vi "Write Notification Msg Return Info.vi"(8 "Return Priority (Normal)":T1=enum."Normal", 9 "Datum Name":string, 10 "Message Enqueuer in":refnum<class "Message Enqueuer.lvclass">, 11 "Notification Msg In":refnum<class "Notification Msg.lvclass">) -> (3 "Notification Msg Out":refnum<class "Notification Msg.lvclass">)   [LabVIEW 2017, in "Transport.lvlib" / "Notification Msg.lvclass"]
doc: "<License>\nCopyright © 2017 Composed Systems, LLC | All rights reserved\nwww.composed.io\n\nAuthor: Ethan Stern <ethan.stern@composed.io>\n\nThis software is provided \"AS IS\" WITHOUT WARRANTIES, either express or implied, AND IS FOR EDUCATIONAL PURPOSES ONLY.\n</License>"
uses:
  Notification Msg.lvclass
  <vilib>/ActorFramework/Message Enqueuer/Message Enqueuer.lvclass
  gpm_packages/@cs/transport/Source/Concrete/ActorMessageTransport/Notification Msg/Notification Msg.lvclass
  <vilib>/ActorFramework/Message Enqueuer/Message Priority.ctl
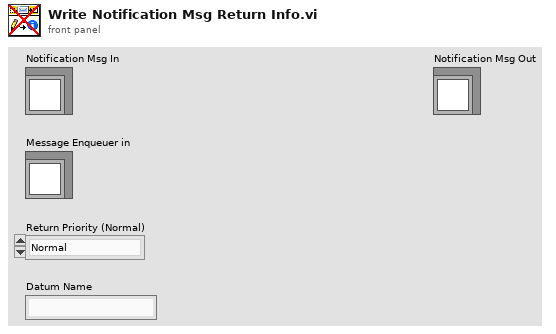
[diagram p1: front panel]
types:
  T1 = typedef "Actor Framework.lvlib/Message Enqueuer.lvclass/Message Priority.ctl" = enum16{"Low", "Normal", "High"}
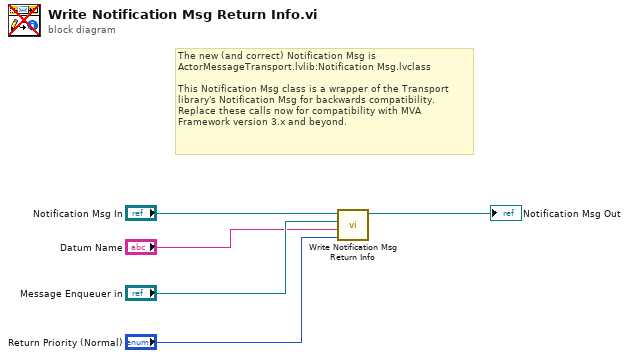
[diagram p0: block diagram]
diagram:
  # "The new (and correct) Notification Msg is\nActorMessageTransport.lvlib:Notification Msg.lvclass\n\nThis Notification Msg class is a wrapper of the Transport\nlibrary's Notification Msg for backwards compatibility.\nReplace these calls now for compatibility with MVA\nFramework version 3.x and beyond."
  n1 = call-parent "Write Notification Msg Return Info.vi"("Return Priority (Normal)"="Return Priority (Normal)", "Datum Name"="Datum Name", "Message Enqueuer in"="Message Enqueuer in", "Notification Msg In"="Notification Msg In") -> ("Notification Msg Out"=→"Notification Msg Out":refnum<class "Notification Msg.lvclass">)  [unwired: 7 in]
